vi "PXI-Synchronize Tasks 2.vi"(0 "Task Specification Array":T1[](array[typedef]) {"Channels"."Terminal configuration" items=["Default"=-1, "RSE"=10083, "Differential"=10106, "Pseudodifferential"=12529]}, 11 "error in (no error)":errorcluster) -> (4 "Task Specification Array Out":T1[](array[typedef]) {"Channels"."Terminal configuration" items=["Default"=-1, "RSE"=10083, "Differential"=10106, "Pseudodifferential"=12529]}, 15 "error out":errorcluster)   [LabVIEW 2020]
uses:
  Type Defs/Task Specification Struct.ctl
  Type Defs/Channel Struct.ctl
  <vilib>/DAQmx/configure/trigger.llb/DAQmx Start Trigger (Digital Edge).vi
  PXI Globals.vi
  <resource>/objmgr/daqmx.rc
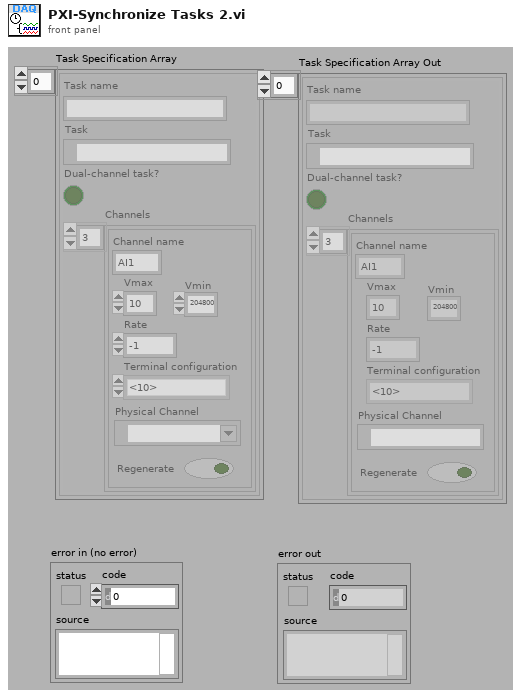
[diagram p1: front panel]
types:
  T1 = typedef "Task Specification Struct.ctl" = cluster{"Task name":string, "Task":refnum<k21>, "Dual-channel task?":bool, "Channels":T2[]}
  T2 = typedef "Channel Struct.ctl" = cluster{"Channel name":string, "Vmax":dbl, "Vmin":dbl, "Rate":dbl, "Terminal configuration":i32, "Physical Channel":tag, "Regenerate":bool}
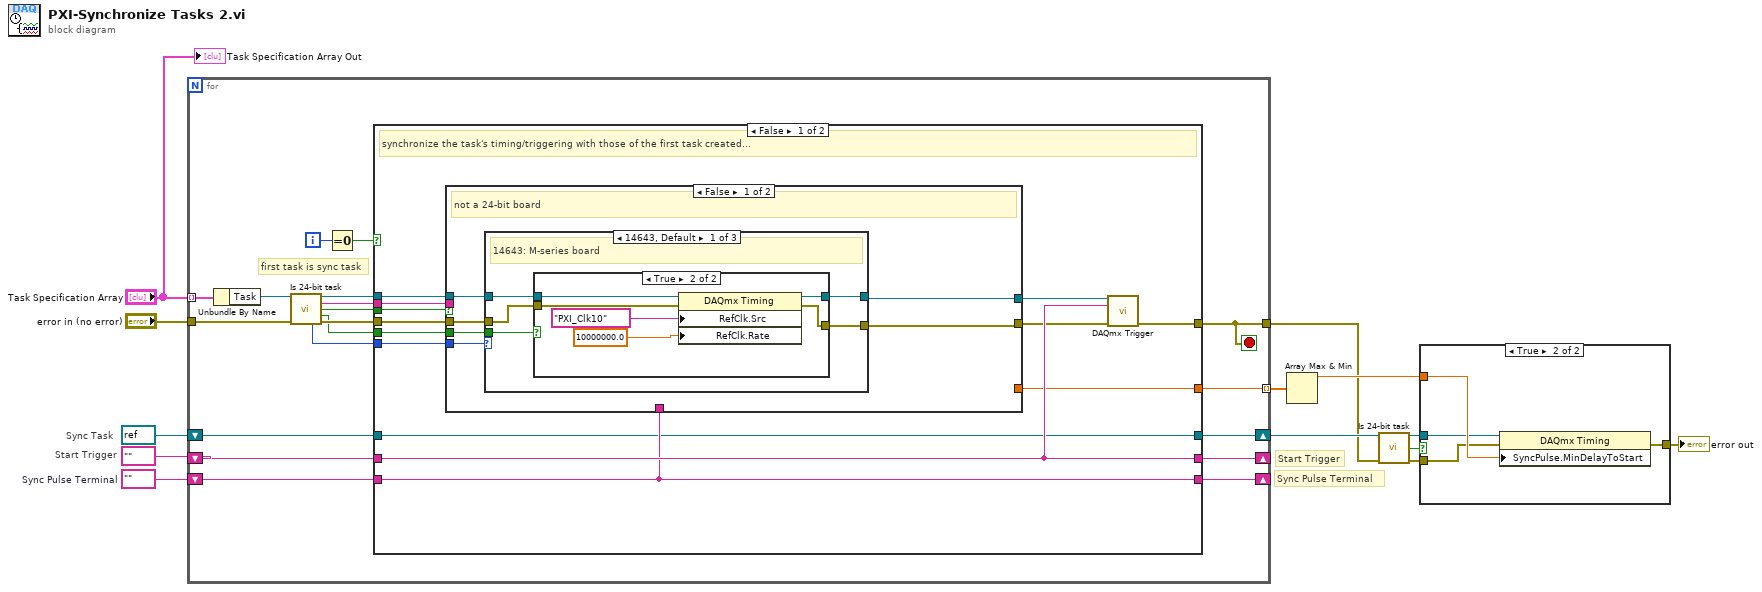
[diagram p0: block diagram]
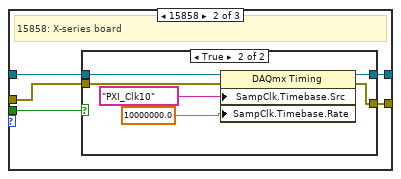
[diagram p4: hidden frame]
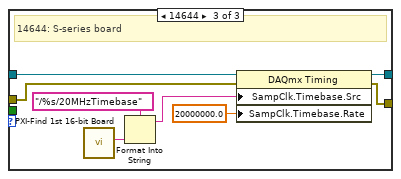
[diagram p6: hidden frame]
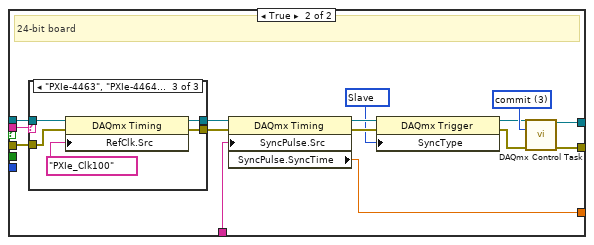
[diagram p7: hidden frame]
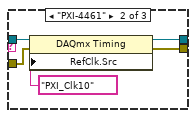
[diagram p9: hidden frame]
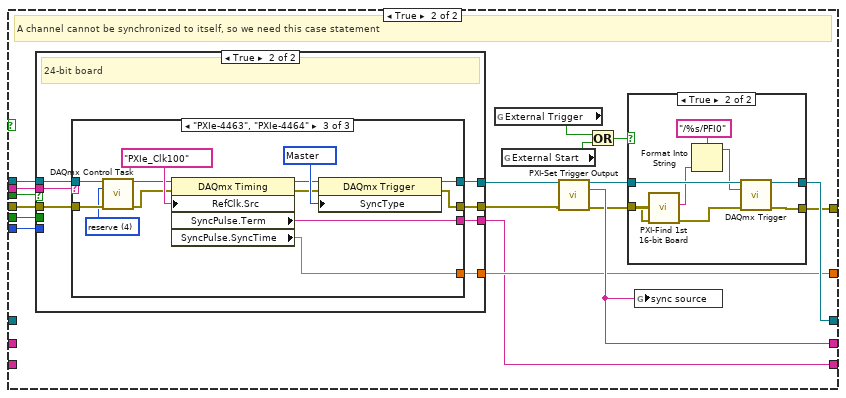
[diagram p10: hidden frame]
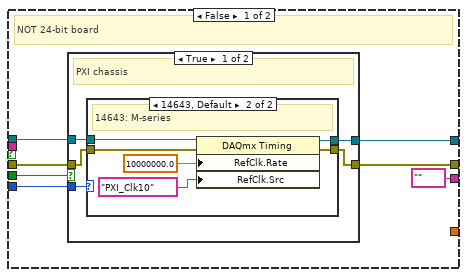
[diagram p11: hidden frame]
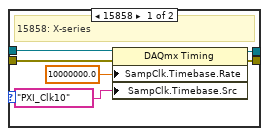
[diagram p12: hidden frame]
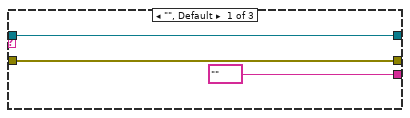
[diagram p14: hidden frame]
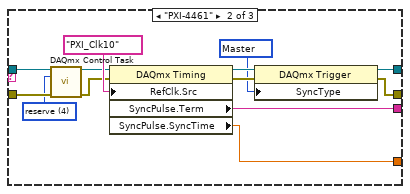
[diagram p15: hidden frame]
diagram:
  w11 = tag ""  # Sync Pulse Terminal
  # "Sync Pulse Terminal"
  # "Start Trigger"
  # "Start Trigger"
  # "Sync Task"
  n1 = for {
    tunnel: "Task Specification Array" -> [w24] mode=indexing
    shift-right: [w32] -> w5
    shift-left: refnum<k21> refnum ("task out") -> [w31]
    shift-right: [w29] -> _
    shift-left: tag "" ("source") -> [w28]
    shift-right: [w27] -> _
    shift-left: w11 -> [w25]
    tunnel: "error in (no error)" -> [w15]
    tunnel: [w20] -> w3
    tunnel: [w14] -> w7 mode=indexing
    i -> [w30]
    stop <- w20 stop-if-true
    # "first task is sync task"
    n2 = Unbundle By Name(w24) -> ("Task"=w16:refnum<k21>)
    n3 = call "Is 24-bit task.vi"("task"=w16, "error in (no error)"=w15) -> ("task out"=w22:refnum<k21>, "Product Type"=w17:string, "is 24bit?"=w19:bool, "PXI?"=w18:bool, "Product Category"=w21:i32, "error out"=w23:errorcluster)  [unwired: 8 in]
    n4 = Equal To 0?(x=w30) -> (x = 0?=w26:bool)
    n5 = case shown="False" w26 {
      tunnel: w23 -> [w43 w122]
      tunnel: [w45 w129] -> w20
      tunnel: [w37 w130] -> w32
      tunnel: w31 -> [w37 _]
      tunnel: [w44 w126] -> w29
      tunnel: w28 -> [w44 _]
      tunnel: [w42 w113] -> w27
      tunnel: w25 -> [w42 _]
      tunnel: w22 -> [w38 w123]
      tunnel: w19 -> [w39 w121]
      tunnel: w21 -> [w36 w120]
      tunnel: w18 -> [w35 w119]
      tunnel: w17 -> [w34 w115]
      tunnel: [w33 w114] -> w14
      frame False {
        # "synchronize the task's timing/triggering with those of the first task created..."
        n6 = case shown="False" w39 {
          tunnel: [w49 w86] -> w41
          tunnel: [w50 w89] -> w40
          tunnel: w43 -> [w47 w100]
          tunnel: w42 -> [_ w99]
          tunnel: w38 -> [w48 w96]
          tunnel: w36 -> [w51 _]
          tunnel: w35 -> [w46 _]
          tunnel: w34 -> [_ w95]
          tunnel: [_ w94] -> w33
          frame False {
            # "not a 24-bit board"
            n7 = case shown="14643, Default" w51 {
              tunnel: [w56 w69 w85] -> w49
              tunnel: [w55 w68 w84] -> w50
              tunnel: w48 -> [w54 w67 w82]
              tunnel: w47 -> [w53 w66 w81]
              tunnel: w46 -> [w52 w65 _]
              frame 14643, Default {
                # "14643: M-series board"
                n8 = case shown="True" w52 {
                  tunnel: [w58 w64] -> w56
                  tunnel: [w57 w63] -> w55
                  tunnel: w54 -> [w58 w60]
                  tunnel: w53 -> [w57 w59]
                  frame False {
                  }
                  frame True {
                    n9 = property class="DAQmx Timing"(reference=w60, error in=w59, "RefClk.Src"=tag "PXI_Clk10", "RefClk.Rate"=10000000.0) -> (reference out=w64:refnum<k21>, error out=w63:errorcluster)
                  }
                }
              }
              frame 15858 {
                # "15858: X-series board"
                n10 = case shown="True" w65 {
                  tunnel: [w71 w77] -> w69
                  tunnel: [w70 w76] -> w68
                  tunnel: w67 -> [w71 w73]
                  tunnel: w66 -> [w70 w72]
                  frame False {
                  }
                  frame True {
                    n11 = property class="DAQmx Timing"(reference=w73, error in=w72, "SampClk.Timebase.Src"=tag "PXI_Clk10" ("RefClk.Src"), "SampClk.Timebase.Rate"=10000000.0) -> (reference out=w77:refnum<k21>, error out=w76:errorcluster)
                  }
                }
              }
              frame 14644 {
                # "14644: S-series board"
                n12 = call "PXI-Find 1st 16-bit Board.vi"() -> ("DAQmx Device Name"=w78:tag)  [unwired: 9 in, 2 out]
                n13 = Format Into String(format string="/%s/20MHzTimebase", w78) -> (resulting string=w79:string)  [unwired: 2 in, 1 out]
                n14 = property class="DAQmx Timing"(reference=w82, error in=w81, "SampClk.Timebase.Src"=w79, "SampClk.Timebase.Rate"=20000000.0) -> (reference out=w85:refnum<k21>, error out=w84:errorcluster)
              }
            }
          }
          frame True {
            w88 = 3 items=["verify"=2, "reserve"=4, "commit"=3, "unreserve"=5, "abort"=6] ("action")
            w91 = 15889 items=["None"=10230, "Master"=15888, "Slave"=15889] ("SyncType")
            # "24-bit board"
            n15 = case shown="\"PXIe-4463\", \"PXIe-4464\"" w95 {
              tunnel: w100 -> [w101 w107 w112]
              tunnel: [w101 w106 w111] -> w98
              tunnel: [w102 w105 w110] -> w97
              tunnel: w96 -> [w102 w104 w109]
              frame "", Default {
              }
              frame "PXI-4461" {
                n16 = property class="DAQmx Timing"(reference=w104, error in=w107, "RefClk.Src"=tag "PXI_Clk10") -> (reference out=w105:refnum<k21>, error out=w106:errorcluster)
              }
              frame "PXIe-4463", "PXIe-4464" {
                n17 = property class="DAQmx Timing"(reference=w109, error in=w112, "RefClk.Src"=tag "PXIe_Clk100") -> (reference out=w110:refnum<k21>, error out=w111:errorcluster)
              }
            }
            n18 = property class="DAQmx Timing"(reference=w97, error in=w98, "SyncPulse.Src"=w99) -> (reference out=w93:refnum<k21>, error out=w92:errorcluster, "SyncPulse.SyncTime"=w94:dbl)
            n19 = property class="DAQmx Trigger"(reference=w93, error in=w92, "SyncType"=w91) -> (reference out=w87:refnum<k21>, error out=w90:errorcluster)
            n20 = call <vilib>:"DAQmx Control Task.vi"("task/channels in"=w87, "action"=w88, "error in"=w90) -> ("task out"=w86:refnum<k21>, "error out"=w89:errorcluster)  [unwired: 11 in]
          }
        }
        n21 = call-poly <vilib>:"DAQmx Trigger.vi"("task/channels in"=w41, "source"=w44, "error in"=w40) -> ("error out"=w45:errorcluster)  [unwired: 11 in, 1 out]
      }
      frame True {
        # "A channel cannot be synchronized to itself, so we need this case statement"
        n22 = case shown="True" w121 {
          tunnel: [w136 w163] -> w127
          tunnel: w123 -> [w137 w161]
          tunnel: [w135 w162] -> w128
          tunnel: w122 -> [w134 w160]
          tunnel: w120 -> [w132 _]
          tunnel: w119 -> [w133 _]
          tunnel: w115 -> [_ w159]
          tunnel: [_ w158] -> w114
          tunnel: [tag "" ("Terminal Name with Device Prefix") w157] -> w113
          frame False {
            # "NOT 24-bit board"
            n23 = case shown="True" w133 {
              tunnel: w137 -> [w142 w156]
              tunnel: [w141 w156] -> w136
              tunnel: [w140 w155] -> w135
              tunnel: w134 -> [w139 w155]
              tunnel: w132 -> [w138 _]
              frame True {
                # "PXI chassis"
                n24 = case shown="14643, Default" w138 {
                  tunnel: w142 -> [w148 w154]
                  tunnel: [w147 w153] -> w141
                  tunnel: [w146 w152] -> w140
                  tunnel: w139 -> [w145 w151]
                  frame 15858 {
                    # "15858: X-series"
                    n25 = property class="DAQmx Timing"(reference=w148, error in=w145, "SampClk.Timebase.Rate"=10000000.0, "SampClk.Timebase.Src"=tag "PXI_Clk10" ("RefClk.Src")) -> (reference out=w147:refnum<k21>, error out=w146:errorcluster)
                  }
                  frame 14643, Default {
                    # "14643: M-series"
                    n26 = property class="DAQmx Timing"(reference=w154, error in=w151, "RefClk.Rate"=10000000.0, "RefClk.Src"=tag "PXI_Clk10") -> (reference out=w153:refnum<k21>, error out=w152:errorcluster)
                  }
                }
              }
              frame False {
                # "NOT PXI chassis"
              }
            }
          }
          frame True {
            # "24-bit board"
            n27 = case shown="\"PXIe-4463\", \"PXIe-4464\"" w159 {
              tunnel: [w166 w169 w182] -> w163
              tunnel: [w165 w168 w181] -> w162
              tunnel: w161 -> [w166 w176 w191]
              tunnel: w160 -> [w165 w174 w190]
              tunnel: [_ w178 w186] -> w158
              tunnel: [tag "" ("SyncPulse.Term") w177 w185] -> w157
              frame "", Default {
              }
              frame "PXI-4461" {
                w167 = 15888 items=["None"=10230, "Master"=15888, "Slave"=15889] ("SyncType")
                w172 = 4 items=["verify"=2, "reserve"=4, "commit"=3, "unreserve"=5, "abort"=6] ("action")
                n28 = call <vilib>:"DAQmx Control Task.vi"("task/channels in"=w176, "action"=w172, "error in"=w174) -> ("task out"=w175:refnum<k21>, "error out"=w173:errorcluster)  [unwired: 11 in]
                n29 = property class="DAQmx Timing"(reference=w175, error in=w173, "RefClk.Src"=tag "PXI_Clk10") -> (reference out=w171:refnum<k21>, error out=w170:errorcluster, "SyncPulse.Term"=w177:tag, "SyncPulse.SyncTime"=w178:dbl)
                n30 = property class="DAQmx Trigger"(reference=w171, error in=w170, "SyncType"=w167) -> (reference out=w169:refnum<k21>, error out=w168:errorcluster)
              }
              frame "PXIe-4463", "PXIe-4464" {
                w184 = 15888 items=["None"=10230, "Master"=15888, "Slave"=15889] ("SyncType")
                w187 = 4 items=["verify"=2, "reserve"=4, "commit"=3, "unreserve"=5, "abort"=6] ("action")
                n31 = call <vilib>:"DAQmx Control Task.vi"("task/channels in"=w191, "action"=w187, "error in"=w190) -> ("task out"=w189:refnum<k21>, "error out"=w188:errorcluster)  [unwired: 11 in]
                n32 = property class="DAQmx Timing"(reference=w189, error in=w188, "RefClk.Src"=tag "PXIe_Clk100") -> (reference out=w183:refnum<k21>, error out=w180:errorcluster, "SyncPulse.Term"=w185:tag, "SyncPulse.SyncTime"=w186:dbl)
                n33 = property class="DAQmx Trigger"(reference=w183, error in=w180, "SyncType"=w184) -> (reference out=w182:refnum<k21>, error out=w181:errorcluster)
              }
            }
          }
        }
        n34 = global read "PXI Globals.vi" "External Trigger"() -> (w118:bool)
        n35 = global read "PXI Globals.vi" "External Start"() -> (w117:bool)
        n36 = call "PXI-Set Trigger Output.vi"("Task in"=w127, "error in (no error)"=w128) -> ("Task out"=w124:refnum<k21>, "Trigger Terminal"=w126:tag, "error out"=w125:errorcluster)  [unwired: 11 in]
        n37 = Or(x=w118, y=w117) -> (x .or. y?=w116:bool)
        n38 = case shown="True" w116 {
          tunnel: [w193 w202] -> w129
          tunnel: w124 -> [w194 w201]
          tunnel: w125 -> [w193 w199]
          tunnel: [w194 w200] -> w130
          frame False {
          }
          frame True {
            n39 = call "PXI-Find 1st 16-bit Board.vi"("error in (no error)"=w199) -> ("error out"=w198:errorcluster, "DAQmx Device Name"=w197:tag)  [unwired: 8 in, 1 out]
            n40 = Format Into String(format string="/%s/PFI0", w197) -> (resulting string=w195:string)  [unwired: 2 in, 1 out]
            n41 = call-poly <vilib>:"DAQmx Trigger.vi"("task/channels in"=w201, "source"=w195, "error in"=w198) -> ("task out"=w200:refnum<k21>, "error out"=w202:errorcluster)  [unwired: 11 in]
          }
        }
        n42 = global write "PXI Globals.vi" "sync source"(w126) -> ()
      }
    }
  }
  n43 = Array Max & Min(array=w7) -> (max value=w6:dbl)  [unwired: 3 out]
  n44 = call "Is 24-bit task.vi"("task"=w5, "error in (no error)"=w3) -> ("task out"=w4:refnum<k21>, "is 24bit?"=w1:bool, "error out"=w2:errorcluster)  [unwired: 8 in, 3 out]
  n45 = case shown="True" w1 {
    tunnel: [w203 w207] -> w8
    tunnel: w6 -> [_ w206]
    tunnel: w4 -> [_ w205]
    tunnel: w2 -> [w203 w204]
    frame False {
    }
    frame True {
      n46 = property class="DAQmx Timing"(reference=w205, error in=w204, "SyncPulse.MinDelayToStart"=w206) -> (error out=w207:errorcluster)  [unwired: 1 out]
    }
  }
  "error out" <- w8
  "Task Specification Array Out" <- "Task Specification Array"
